vi "Main.vi"(8 "error in":errorcluster, 11 "Head Worker in":refnum<class "Head Worker.lvclass">) -> (0 "error out":errorcluster, 3 "Head Worker out":refnum<class "Head Worker.lvclass">)   [LabVIEW 2017, in "Head Worker.lvclass"]
doc: "The <b>Queued Message Handler</b> of the Worker that owns this VI."
uses:
  Head Worker.lvclass
  C:/Program Files (x86)/National Instruments/LabVIEW 2017/vi.lib/addons/_Workers/Library/Classes/Worker/Worker.lvclass
  Client Data.ctl
  Head Worker.lvclass/Head Worker.ctl
  Initialization Data.ctl
  TCP Server/TCP Server/rqp_Start Listening.ctl
  TCP Server/TCP Server/rqp_Send String to Clients.ctl
  <vilib>/addons/_Workers/Library/Classes/Message Queue/Message Queue.lvclass
  TCP Server/TCP Server/TCP Server.lvclass
panel:
  in  "Server Name":string="Host TCP Server"
  out "Listening":bool
  in  "Server Port":u16=9123
  in  "Start/Stop Listening":bool caption="Disconnect from Server"
  in  "TCP Client":T1
  # "Server Name"
  # "Server Port"
  # "Client Name :"
  # "IP Address :"
  # "Connected? :"
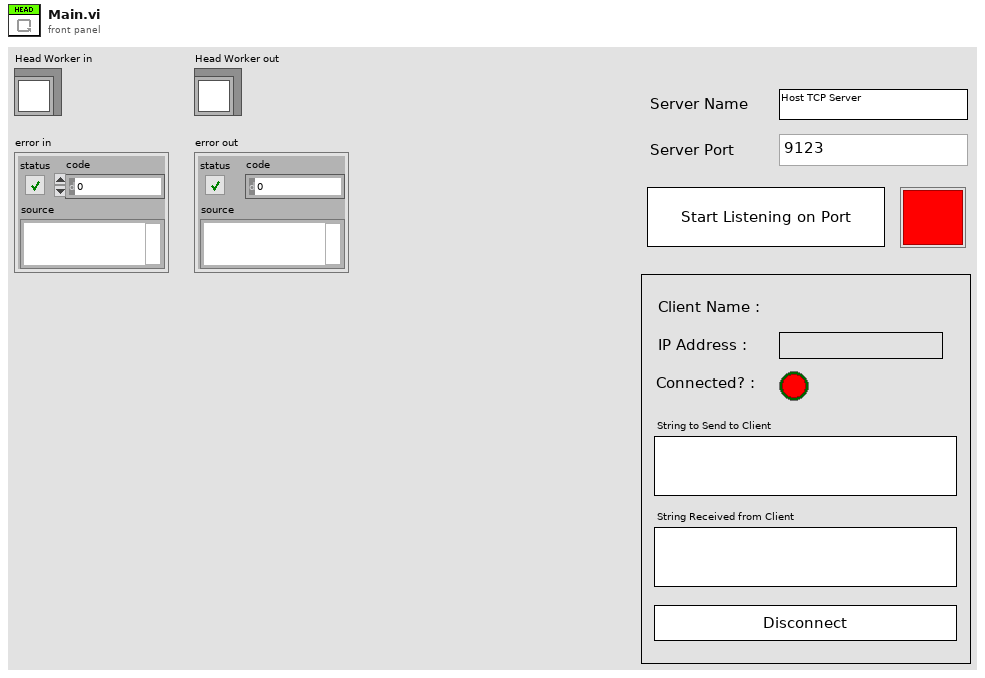
[diagram p1: front panel]
types:
  T1 = typedef "Head Worker.lvclass/Client Data.ctl" = cluster{"Client Name":string, "IP Address":string, "Connected?":bool, "String to Send to Client":string, "String Received from Client":string, "Disconnect from Client":bool}
  T2 = typedef "Head Worker.lvclass/Initialization Data.ctl" = cluster{"String":string}
  T3 = typedef "TCP Server.lvlib/TCP Server.lvclass/rqp_Start Listening.ctl" = cluster{"Server Name":string, "Server IP Address":string, "Server Port":u16}
  T4 = typedef "TCP Server.lvlib/TCP Server.lvclass/rqp_Send String to Clients.ctl" = cluster{"TCP Client Names":string[], "String to Send":string}
  T5 = typedef "TCP Server.lvlib/TCP Server.lvclass/rsp_Connection Notify.ctl" = cluster{"Client Name":string, "IP Address":string, "Connected?":bool}
  T6 = typedef "TCP Server.lvlib/TCP Server.lvclass/rsp_Incoming Data.ctl" = cluster{"Client Name":string, "Data":string}
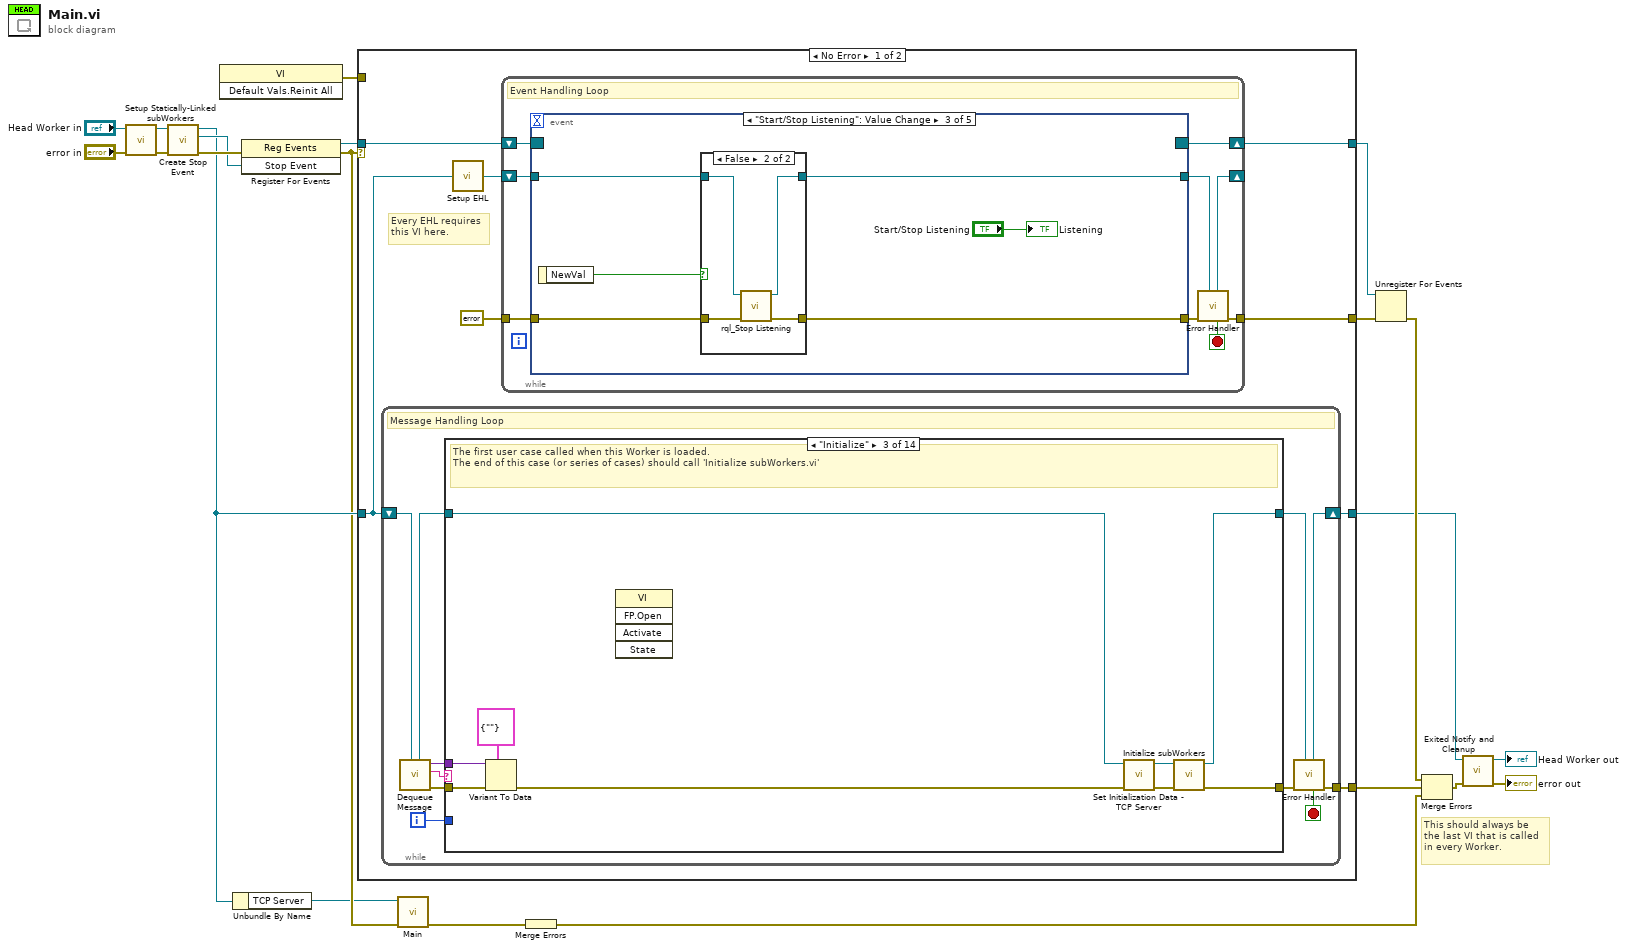
[diagram p0: block diagram]
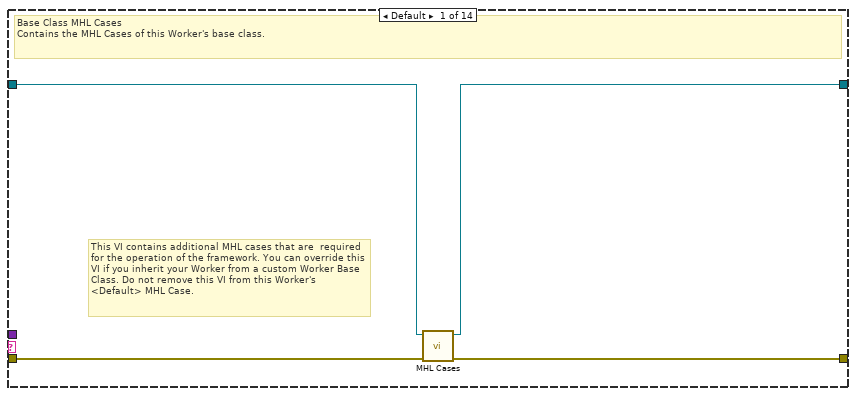
[diagram p2: hidden frame]
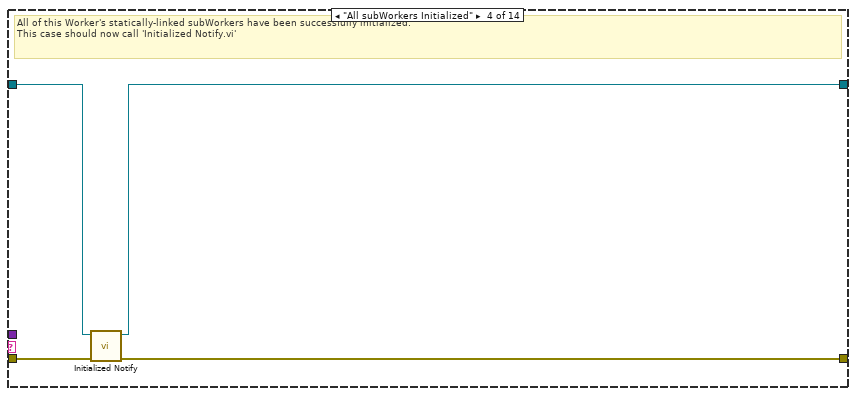
[diagram p4: hidden frame]
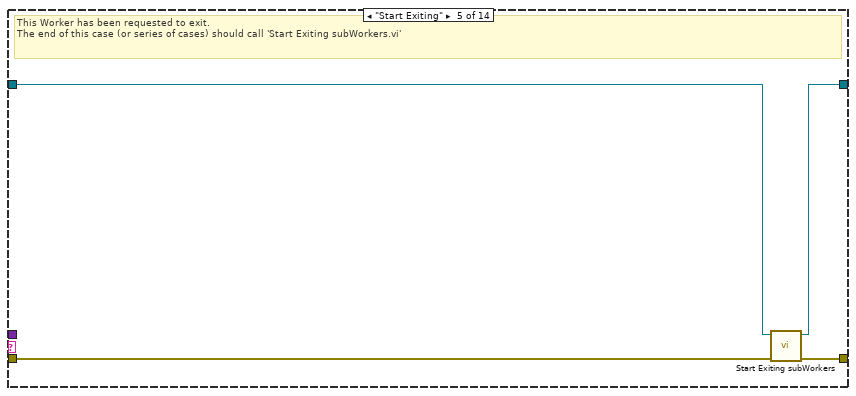
[diagram p5: hidden frame]
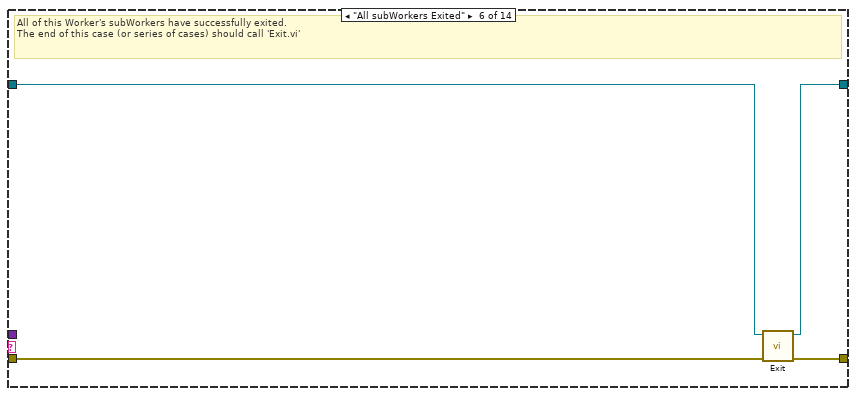
[diagram p6: hidden frame]
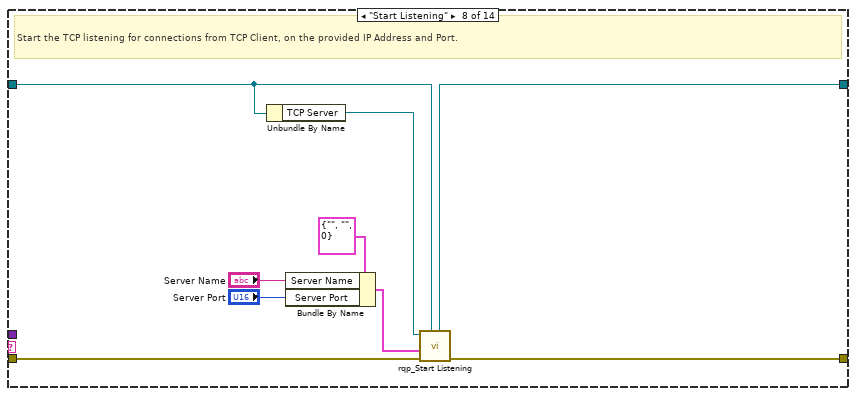
[diagram p8: hidden frame]
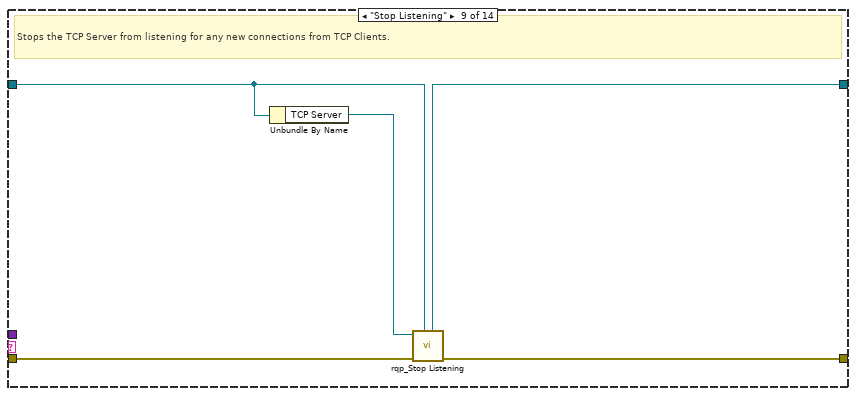
[diagram p9: hidden frame]
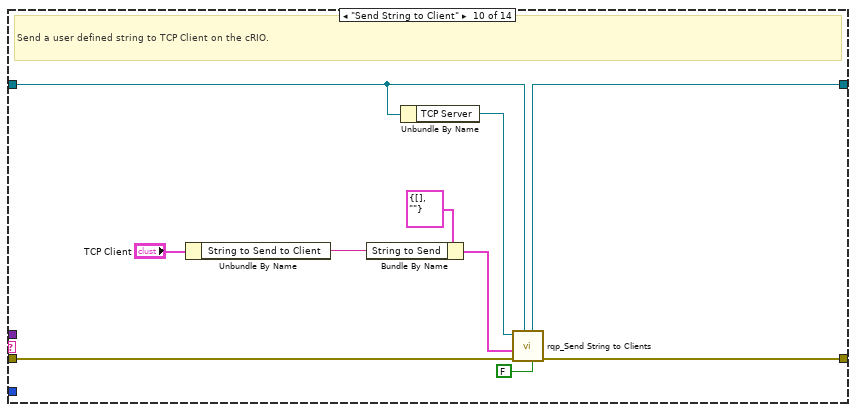
[diagram p10: hidden frame]
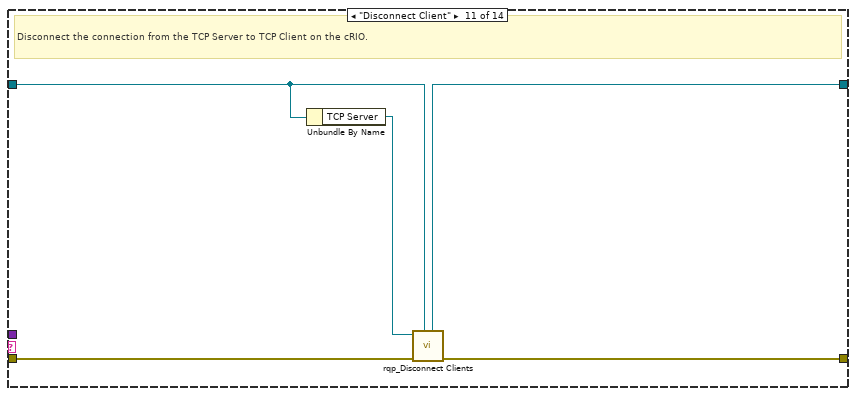
[diagram p11: hidden frame]
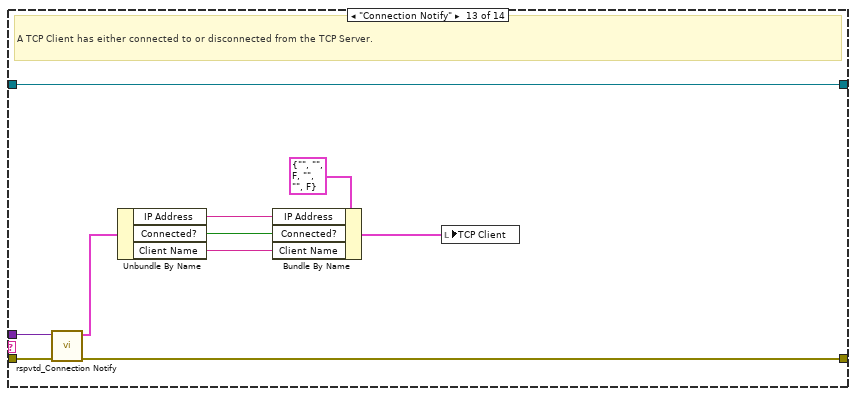
[diagram p13: hidden frame]
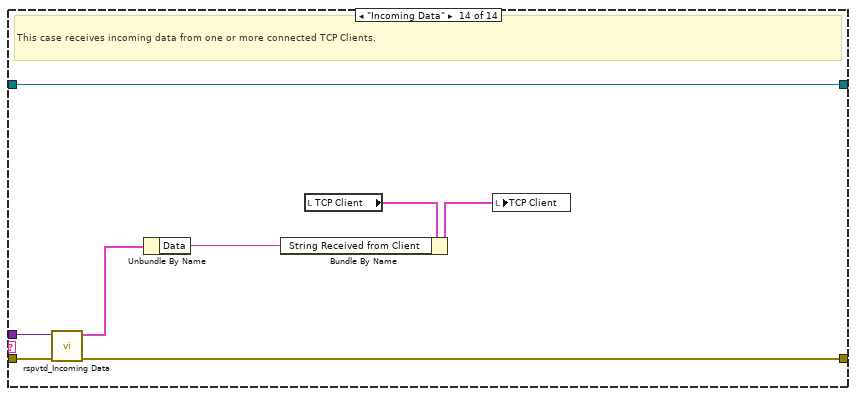
[diagram p14: hidden frame]
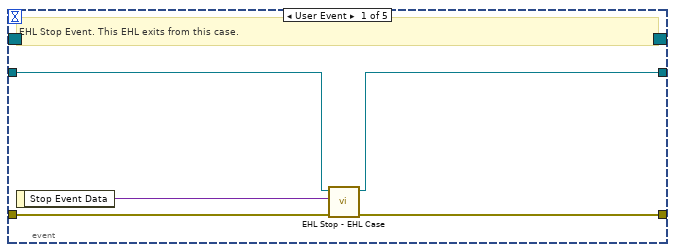
[diagram p15: hidden frame]
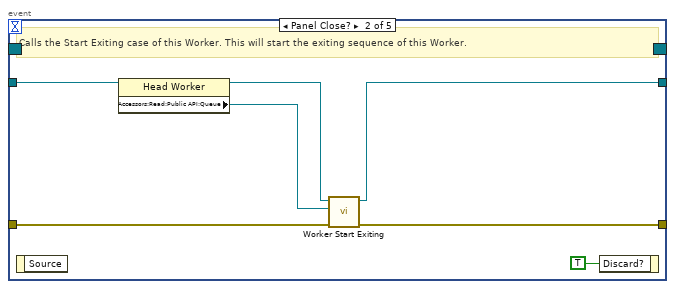
[diagram p16: hidden frame]
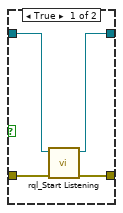
[diagram p17: hidden frame]
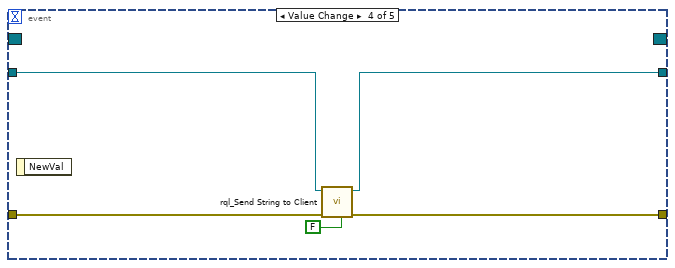
[diagram p18: hidden frame]
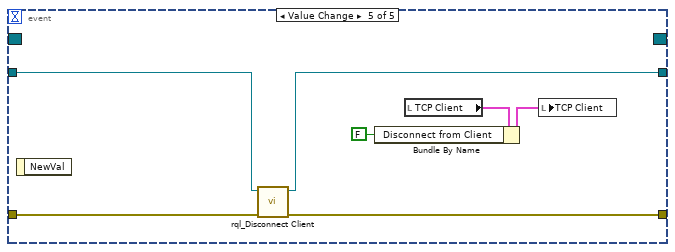
[diagram p19: hidden frame]
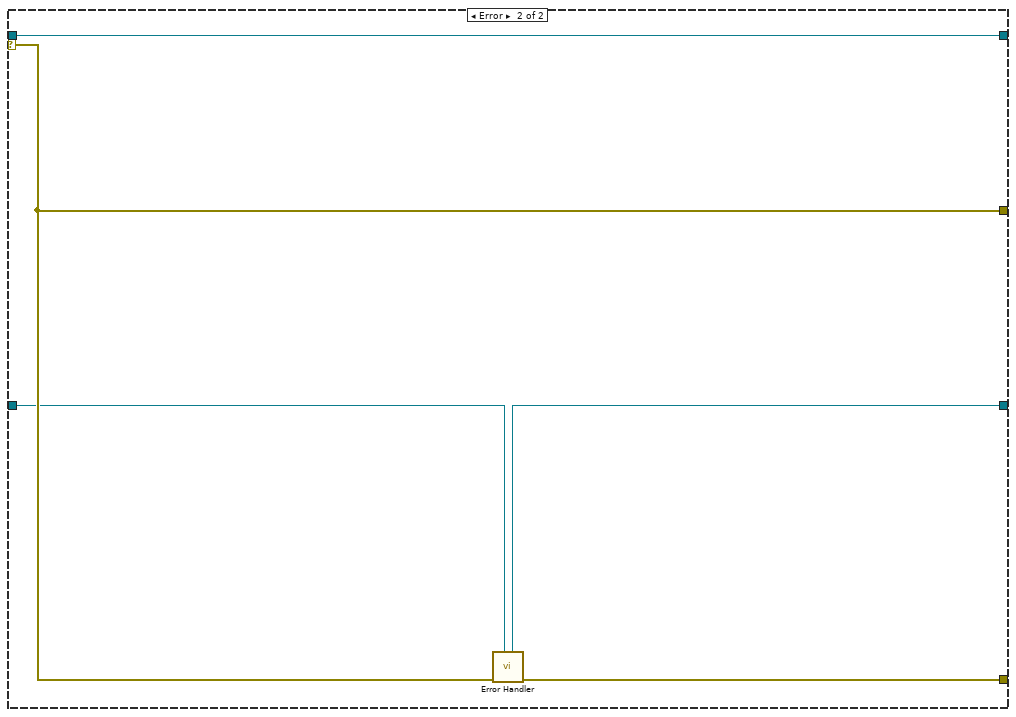
[diagram p20: hidden frame]
diagram:
  # "This should always be the last VI that is called in every Worker."
  n1 = call "Setup Statically-Linked subWorkers.vi"("error in"="error in", "Head Worker in"="Head Worker in") -> ("error out"=w6:errorcluster, "Head Worker out"=w4:refnum<class "Head Worker.lvclass">)  [unwired: 8 in]
  n2 = call-dynamic "Create Stop Event.vi"("error in"=w6, "Worker"=w4) -> ("error out"=w16:errorcluster, "Stop Event"=w13:refnum<user-event>, "Worker out"=w10:refnum<class "Head Worker.lvclass">)  [unwired: 7 in]
  n3 = invoke class="VI" method="Default Vals.Reinit All"() -> (error out=w8:errorcluster)  [unwired: 3 in, 2 out]
  n4 = Unbundle By Name(w10) -> ("TCP Server"=w1:refnum<class "TCP Server.lvclass">)
  n5 = register-events(error in=w16, w13) -> (reference out=w15:refnum<event-registration>, error out=w9:errorcluster)  [unwired: 1 in]
  n6 = case shown="No Error" w9 {
    tunnel: w10 -> [w24 w167]
    tunnel: [w22 w168] -> w14
    tunnel: w15 -> [w29 w169]
    tunnel: [w26 w170] -> w20
    tunnel: [w28 w169] -> w19
    tunnel: [w23 w166] -> w17
    selector: w9 -> [_ w170]
    tunnel: w8 -> [_ _]
    frame No Error {
      # "Every EHL requires\nthis VI here."
      n7 = while {
        shift-right: [w38] -> w23
        shift-left: w24 -> [w40]
        tunnel: [w39] -> w22
        i -> [w31]
        stop <- w32 stop-if-true
        # "Message Handling Loop"
        n8 = call-dynamic "Dequeue Message.vi"("Worker"=w40) -> ("error out"=w37:errorcluster, "Case out"=w33:string, "Data out"=w30:variant, "Worker out"=w35:refnum<class "Head Worker.lvclass">)  [unwired: 6 in, 1 out]
        n9 = case "Worker MHL Case Structure (DO NOT CHANGE LABEL NAME)" shown="\"Initialize\"" w33 {
          tunnel: w37 -> [w44 w45 w53 w58 w60 w67 w69 w78 w83 w93 w98 w100 w110 w118]
          tunnel: [w43 w45 w55 w56 w63 w66 w69 w77 w82 w92 w97 w100 w108 w116] -> w36
          tunnel: w35 -> [w42 w46 w47 w59 w61 w65 w68 w71 w80 w89 w95 w99 w109 w117]
          tunnel: [w41 w46 w54 w57 w62 w64 w68 w76 w81 w91 w96 w99 w109 w117] -> w34
          tunnel: w31 -> [_ _ _ _ _ _ _ _ _ _ _ _ _ _]
          tunnel: w30 -> [_ _ w51 _ _ _ _ _ _ _ _ _ w107 w115]
          frame Default {
            # "This VI contains additional MHL cases that are  required for the operation of the framework. You can override this VI if you inherit your Worker from a custom Worker Base Class. Do not remove this VI from this Worker's <Default> MHL Case."
            # "Base Class MHL Cases\nContains the MHL Cases of this Worker's base class."
            n10 = call-dynamic "MHL Cases.vi"("error in"=w44, "Worker in"=w42) -> ("error out"=w43:errorcluster, "Worker out"=w41:refnum<class "Head Worker.lvclass">)  [unwired: 8 in]
          }
          frame "------------ FRAMEWORK CASES -----------" {
            # "Start of Workers Framework Cases"
          }
          frame "Initialize" {
            # "The first user case called when this Worker is loaded.\nThe end of this case (or series of cases) should call 'Initialize subWorkers.vi'"
            n11 = Variant To Data(error in=w53, type=T2 {"String"=""} ("Initialization Data"), Variant=w51) -> (error out=w52:errorcluster)  [unwired: 1 out]
            n12 = invoke class="VI" method="FP.Open"() -> ()  [unwired: 5 in, 5 out]
            n13 = call "Set Initialization Data - TCP Server.vi"("error in"=w52, "Head Worker in"=w47) -> ("error out"=w49:errorcluster, "Head Worker out"=w48:refnum<class "Head Worker.lvclass">)  [unwired: 8 in]
            n14 = call-dynamic "Initialize subWorkers.vi"("error in"=w49, "Worker"=w48) -> ("error out"=w55:errorcluster, "dup Worker out"=w54:refnum<class "Head Worker.lvclass">)  [unwired: 8 in]
          }
          frame "All subWorkers Initialized" {
            # "All of this Worker's statically-linked subWorkers have been successfully initialized.\nThis case should now call 'Initialized Notify.vi'"
            n15 = call-dynamic "Initialized Notify.vi"("error in"=w58, "Worker"=w59) -> ("error out"=w56:errorcluster, "dup Worker out"=w57:refnum<class "Head Worker.lvclass">)  [unwired: 8 in]
          }
          frame "Start Exiting" {
            # "This Worker has been requested to exit. \nThe end of this case (or series of cases) should call 'Start Exiting subWorkers.vi'"
            n16 = call-dynamic "Start Exiting subWorkers.vi"("error_in"=w60, "Worker"=w61) -> ("error out"=w63:errorcluster, "dup Worker out"=w62:refnum<class "Head Worker.lvclass">)  [unwired: 8 in]
          }
          frame "All subWorkers Exited" {
            # "All of this Worker's subWorkers have successfully exited. \nThe end of this case (or series of cases) should call 'Exit.vi'"
            n17 = call-dynamic "Exit.vi"("error_in"=w67, "Worker"=w65) -> ("error out"=w66:errorcluster, "dup Worker out"=w64:refnum<class "Head Worker.lvclass">)  [unwired: 8 in]
          }
          frame "------------- LOCAL API CASES -------------" {
            # "Start of Workers Local API Cases"
          }
          frame "Start Listening" {
            # "Start the TCP listening for connections from TCP Client, on the provided IP Address and Port."
            n18 = Unbundle By Name(w71) -> ("TCP Server"=w70:refnum<class "TCP Server.lvclass">)
            n19 = Bundle By Name(cluster=T3 {"Server Name"="", "Server IP Address"="", "Server Port"=0} ("Data"), "Server Name"="Server Name", "Server Port"="Server Port") -> (w74:T3)
            n20 = call "rqp_Start Listening.vi"("Caller in"=w71, "error in"=w78, "Data in"=w74, "TCP Server in"=w70) -> ("error out"=w77:errorcluster, "dup Caller out"=w76:refnum<class "Head Worker.lvclass">)  [unwired: 5 in, 1 out]
          }
          frame "Stop Listening" {
            # "Stops the TCP Server from listening for any new connections from TCP Clients."
            n21 = Unbundle By Name(w80) -> ("TCP Server"=w79:refnum<class "TCP Server.lvclass">)
            n22 = call "rqp_Stop Listening.vi"("Caller in"=w80, "error in"=w83, "TCP Server in"=w79) -> ("error out"=w82:errorcluster, "dup Caller out"=w81:refnum<class "Head Worker.lvclass">)  [unwired: 6 in, 1 out]
          }
          frame "Send String to Client" {
            # "Send a user defined string to TCP Client on the cRIO."
            n23 = Unbundle By Name("TCP Client") -> ("String to Send to Client"=w85:string)
            n24 = Bundle By Name(cluster=T4 {"TCP Client Names"=[], "String to Send"=""} ("Data in"), "String to Send"=w85) -> (w86:T4)
            n25 = Unbundle By Name(w89) -> ("TCP Server"=w88:refnum<class "TCP Server.lvclass">)
            n26 = call "rqp_Send String to Clients.vi"("Show in Debugger?"=FALSE, "Caller in"=w89, "error in"=w93, "Data in"=w86, "TCP Server in"=w88) -> ("error out"=w92:errorcluster, "dup Caller out"=w91:refnum<class "Head Worker.lvclass">)  [unwired: 4 in, 1 out]
          }
          frame "Disconnect Client" {
            # "Disconnect the connection from the TCP Server to TCP Client on the cRIO."
            n27 = Unbundle By Name(w95) -> ("TCP Server"=w94:refnum<class "TCP Server.lvclass">)
            n28 = call "rqp_Disconnect Clients.vi"("Caller in"=w95, "error in"=w98, "TCP Server in"=w94) -> ("error out"=w97:errorcluster, "dup Caller out"=w96:refnum<class "Head Worker.lvclass">)  [unwired: 6 in, 1 out]
          }
          frame "------------- RESPONSE CASES --------------" {
            # "Start of Workers Response Cases"
          }
          frame "Connection Notify" {
            # "A TCP Client has either connected to or disconnected from the TCP Server."
            n29 = call "rspvtd_Connection Notify.vi"("error in"=w110, "Data in"=w107) -> ("error out"=w108:errorcluster, "Data out"=w106:T5)  [unwired: 8 in]
            n30 = Unbundle By Name(w106) -> ("IP Address"=w103:string, "Connected?"=w104:bool, "Client Name"=w102:string)
            n31 = Bundle By Name(cluster=T1 {"Client Name"="", "IP Address"="", "Connected?"=FALSE, "String to Send to Client"="", "String Received from Client"="", "Disconnect from Client"=FALSE} ("Client Connection 1"), "IP Address"=w103, "Connected?"=w104, "Client Name"=w102) -> (w101:T1)
            n32 = local write "TCP Client"(w101) -> ()
          }
          frame "Incoming Data" {
            # "This case receives incoming data from one or more connected TCP Clients."
            n33 = call "rspvtd_Incoming Data.vi"("error in"=w118, "Data in"=w115) -> ("error out"=w116:errorcluster, "Data out"=w114:T6)  [unwired: 8 in]
            n34 = Unbundle By Name(w114) -> ("Data"=w113:string)
            n35 = local read "TCP Client"() -> (w112:T1)
            n36 = Bundle By Name(cluster=w112, "String Received from Client"=w113) -> (w111:T1)
            n37 = local write "TCP Client"(w111) -> ()
          }
        }
        n38 = call-dynamic "Error Handler.vi"("Worker"=w34, "error_in"=w36) -> ("error out"=w39:errorcluster, "Stop Loop"=w32:bool, "Worker out"=w38:refnum<class "Head Worker.lvclass">)  [unwired: 7 in]
      }
      n39 = call-dynamic "Setup EHL.vi"("Worker"=w24) -> ("Worker out"=w25:refnum<class "Head Worker.lvclass">)  [unwired: 14 in]
      n40 = while "Event Handling Loop" {
        shift-right: [w127] -> w28
        shift-left: w29 -> [w126]
        tunnel: [w122] -> w26
        tunnel: errorcluster {"status"=FALSE, "code"=0, "source"=""} ("error constant") -> [w124]
        shift-right: [w120] -> _
        shift-left: w25 -> [w125]
        stop <- w119 stop-if-true
        # "Event Handling Loop"
        n41 = event shown="[2] \"Start/Stop Listening\": Value Change" {
          selector: w126 -> [_ _ _ _ _]
          dyn-events: [_ _ _ _ _] -> w127
          timeout: _ -> [_ _ _ _ _]
          tunnel: [w131 w138 w143 w157 w161] -> w123
          tunnel: w124 -> [w132 w137 w145 w158 w165]
          tunnel: w125 -> [w130 w136 w142 w156 w160]
          tunnel: [w129 w135 w141 w155 w159] -> w121
          event User Event {
            # "EHL Stop Event. This EHL exits from this case."
            n42 = event-data() -> ("Stop Event Data"=w128:variant)  [unwired: 1 in]
            n43 = call-dynamic "EHL Stop - EHL Case.vi"("error in"=w132, "Stop Event Data"=w128, "Worker"=w130) -> ("error out"=w131:errorcluster, "Worker out"=w129:refnum<class "Head Worker.lvclass">)  [unwired: 7 in]
          }
          event Panel Close? {
            # "Calls the Start Exiting case of this Worker. This will start the exiting sequence of this Worker."
            n44 = event-data() -> ()  [unwired: 1 in, 1 out]
            n45 = property class="Head Worker"(reference=w136) -> (reference out=w134:refnum<class "Head Worker.lvclass">, "Accessors:Read:Public API:Queue"=w133:refnum<class "Message Queue.lvclass">)  [unwired: 1 in, 1 out]
            n46 = call-dynamic "Worker Start Exiting.vi"("error_in"=w137, "Message Queue"=w133, "Worker"=w134) -> ("error out"=w138:errorcluster, "dup Worker out"=w135:refnum<class "Head Worker.lvclass">)  [unwired: 7 in]
            n47 = event-data ("Event Filter Node")("Discard?"=TRUE) -> ()  [unwired: 1 in, 1 out]
          }
          event "Start/Stop Listening": Value Change {
            n48 = event-data() -> ("NewVal"=w140:bool)  [unwired: 1 in]
            n49 = case shown="False" w140 {
              tunnel: w145 -> [w149 w153]
              tunnel: [w148 w152] -> w143
              tunnel: w142 -> [w147 w151]
              tunnel: [w146 w150] -> w141
              frame True {
                n50 = call "rql_Start Listening.vi"("error in"=w149, "Head Worker in"=w147) -> ("error out"=w148:errorcluster, "dup Head Worker out"=w146:refnum<class "Head Worker.lvclass">)  [unwired: 8 in]
              }
              frame False {
                n51 = call "rql_Stop Listening.vi"("error in"=w153, "Head Worker in"=w151) -> ("error out"=w152:errorcluster, "dup Head Worker out"=w150:refnum<class "Head Worker.lvclass">)  [unwired: 8 in]
              }
            }
            "Listening" <- "Start/Stop Listening"
          }
          event Value Change {
            n52 = event-data() -> ()  [unwired: 1 in, 1 out]
            n53 = call "rql_Send String to Client.vi"("Show in Debugger?"=FALSE, "error in"=w158, "Head Worker in"=w156) -> ("error out"=w157:errorcluster, "dup Head Worker out"=w155:refnum<class "Head Worker.lvclass">)  [unwired: 7 in]
          }
          event Value Change {
            n54 = event-data() -> ()  [unwired: 1 in, 1 out]
            n55 = call "rql_Disconnect Client.vi"("error in"=w165, "Head Worker in"=w160) -> ("error out"=w161:errorcluster, "dup Head Worker out"=w159:refnum<class "Head Worker.lvclass">)  [unwired: 8 in]
            n56 = local read "TCP Client"() -> (w162:T1)
            n57 = Bundle By Name(cluster=w162, "Disconnect from Client"=FALSE ("Connected?")) -> (w164:T1)
            n58 = local write "TCP Client"(w164) -> ()
          }
        }
        n59 = call-dynamic "Error Handler.vi"("Worker"=w121, "error_in"=w123) -> ("error out"=w122:errorcluster, "Stop Loop"=w119:bool, "Worker out"=w120:refnum<class "Head Worker.lvclass">)  [unwired: 7 in]
      }
    }
    frame Error {
      n60 = call-dynamic "Error Handler.vi"("Worker"=w167, "error_in"=w170) -> ("error out"=w168:errorcluster, "Worker out"=w166:refnum<class "Head Worker.lvclass">)  [unwired: 7 in, 1 out]
    }
  }
  n61 = call-dynamic "Main.vi"("error in"=w9, "TCP Server in"=w1) -> ("error out"=w3:errorcluster)  [unwired: 8 in, 1 out]
  n62 = Merge Errors(w3) -> (w2:errorcluster)
  n63 = Unregister For Events(event registration refnum=w19, error in=w20) -> (error out=w21:errorcluster)
  n64 = Merge Errors(w21, w14, w2) -> (w18:errorcluster)
  n65 = call-dynamic "Exited Notify and Cleanup.vi"("error_in"=w18, "Worker"=w17) -> ("error out"=→"error out":errorcluster, "dup Worker out"=→"Head Worker out":refnum<class "Head Worker.lvclass">)  [unwired: 8 in]
